vi "UDS_TimeTips.vi"(8 "error in":errorcluster, 10 "result array":i32[](array[numeric]), 11 "path":path) -> (0 "错误输出":errorcluster, 3 "result":bool)   [LabVIEW 2014]
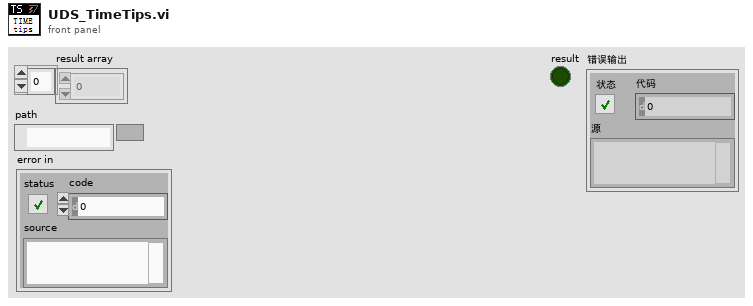
[diagram p1: front panel]
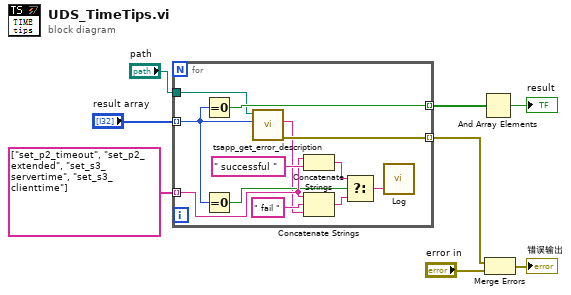
[diagram p0: block diagram]
diagram:
  n1 = for {
    tunnel: "result array" -> [w11] mode=indexing
    tunnel: [w20] -> w8 mode=indexing
    tunnel: "path" -> [w15]
    tunnel: [w14] -> w3 mode=indexing
    tunnel: string[] ["set_p2_timeout", "set_p2_extended", "set_s3_servertime", "set_s3_clienttime"] -> [w12] mode=indexing
    n2 = Equal To 0?(x=w11) -> (x = 0?=w20:bool)
    n3 = Equal To 0?(x=w11) -> (x = 0?=w10:bool)
    n4 = call "tsapp_get_error_description.vi"("ACount"=w11, "路径输入"=w15) -> ("error out"=w14:errorcluster, "ErrDes"=w9:string)  [unwired: 7 in, 1 out]
    n5 = Concatenate Strings(w12, " successful ") -> (w13:string)
    n6 = Concatenate Strings(w12, " fail ", w9) -> (w18:string)
    n7 = Select(t=w13, s=w10, f=w18) -> (s? t:f=w16:string)
    n8 = call "Log.vi"("Data"=w16) -> ()  [unwired: 3 in]
  }
  n9 = And Array Elements(Boolean array=w8) -> (logical AND=→"result":bool)
  n10 = Merge Errors(w3, "error in") -> (→"错误输出":errorcluster)
